vi "FRCts20_Backend_Dyn_FGV.vi"(8 "error in":errorcluster, 9 "VI List":path[](array[path]), 10 "VI to Locate":path, 11 "Command":T1) -> (0 "error out":errorcluster, 1 "VI List Out":path[](array[path]), 2 "vi reference":refnum<vi>)   [LabVIEW 2013, in "FRCts20_Backend_Engine.lvlib"]
uses:
  FRCts20_Backend_Engine.lvlib
  FRCts20_Backend_Dyn_FGV_Command.ctl
  INI_Accessor/FRCts20_Backend_INI Controller.lvclass
  FRCts20_Backend_Dyn_Refnums.ctl
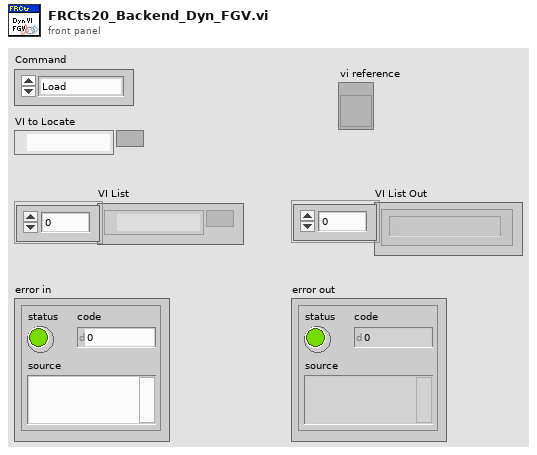
[diagram p1: front panel]
types:
  T1 = typedef "FRCts20_Backend_Engine.lvlib/FRCts20_Backend_Dyn_FGV_Command.ctl" = enum16{"Load", "Locate", "Unload"}
  T2 = typedef "FRCts20_Backend_Engine.lvlib/FRCts20_Backend_Dyn_Refnums.ctl" = cluster{"VI Name":path, "vi reference":refnum<vi>}
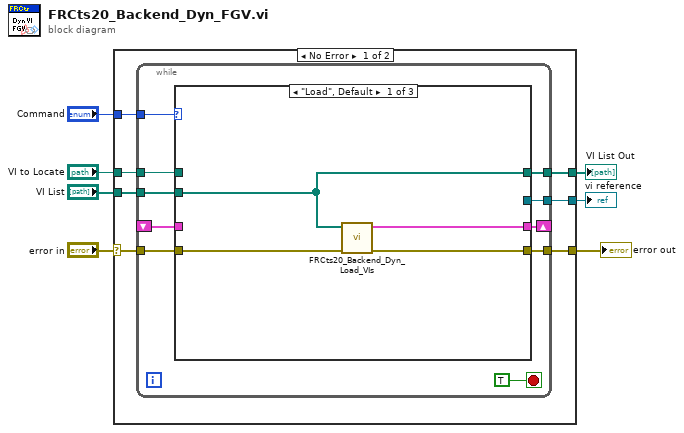
[diagram p0: block diagram]
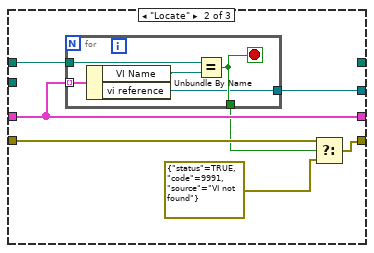
[diagram p2: hidden frame]
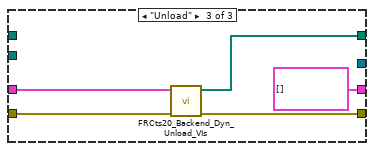
[diagram p3: hidden frame]
diagram:
  n1 = case shown="No Error" "error in" {
    selector: "error in" -> [w9 w47]
    tunnel: "Command" -> [w14 _]
    tunnel: [w13 w47] -> w6
    tunnel: "VI List" -> [w12 w46]
    tunnel: "VI to Locate" -> [w11 _]
    tunnel: [w10 _] -> w1
    tunnel: [w8 w46] -> w2
    frame No Error {
      n2 = while {
        tunnel: w14 -> [w23]
        tunnel: [w22] -> w13
        tunnel: w9 -> [w21]
        shift-right: [w20] -> _
        shift-left: _ -> [w19]
        tunnel: w12 -> [w18]
        tunnel: w11 -> [w17]
        tunnel: [w16] -> w10
        tunnel: [w15] -> w8
        stop <- TRUE stop-if-true
        n3 = case shown="\"Load\", Default" w23 {
          tunnel: w21 -> [w28 w31 w45]
          tunnel: [w27 w32 w42] -> w22
          tunnel: [w26 w33 T2[] [] ("VI Names and Refnums")] -> w20
          tunnel: w19 -> [_ w33 w44]
          tunnel: w18 -> [w25 _ _]
          tunnel: w17 -> [_ w35 _]
          tunnel: [_ w34 _] -> w16
          tunnel: [w25 _ w43] -> w15
          frame "Load", Default {
            n4 = call "FRCts20_Backend_Dyn_Load_VIs.vi"("error in"=w28, "VI Names"=w25) -> ("error out"=w27:errorcluster, "VI Names and Refnums"=w26:T2[])  [unwired: 8 in]
          }
          frame "Locate" {
            n5 = for {
              tunnel: w35 -> [w38]
              tunnel: w33 -> [w40] mode=indexing
              tunnel: [w37] -> w30
              tunnel: [w36] -> w34
              stop <- w37 stop-if-true
              n6 = Unbundle By Name(w40) -> ("VI Name"=w39:path, "vi reference"=w36:refnum<vi>)
              n7 = Equal?(x=w38, y=w39) -> (x = y?=w37:bool)
            }
            n8 = Select(t=w31, s=w30, f=errorcluster {"status"=TRUE, "code"=9991, "source"="VI not found"} ("error constant")) -> (s? t:f=w32:errorcluster)
          }
          frame "Unload" {
            n9 = call "FRCts20_Backend_Dyn_Unload_VIs.vi"("error in"=w45, "VI Names and Refnums"=w44) -> ("error out"=w42:errorcluster, "VI Names"=w43:path[])  [unwired: 8 in]
          }
        }
      }
    }
    frame Error {
    }
  }
  "error out" <- w6
  "VI List Out" <- w2
  "vi reference" <- w1
